vi "Unregister-user-events.vi"(8 "error in (no error)":errorcluster, 10 "Event registration":refnum<event-registration>, 11 "Object ref in":T1) -> (0 "error out":errorcluster, 3 "Object ref out":T1)   [LabVIEW 2013, in "MaterialCharacterization.lvlib" / "MC-Main.lvclass"]
uses:
  MC-Main.lvclass
  Object-reference.ctl
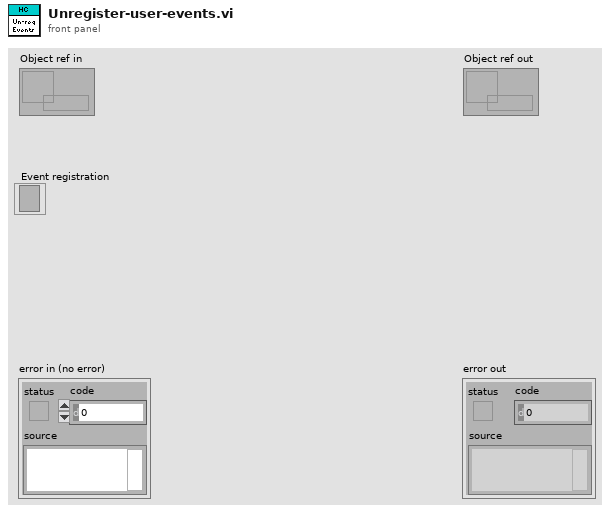
[diagram p1: front panel]
types:
  T1 = typedef "MaterialCharacterization.lvlib/MC-Main.lvclass/Object-reference.ctl" = refnum<data-value>
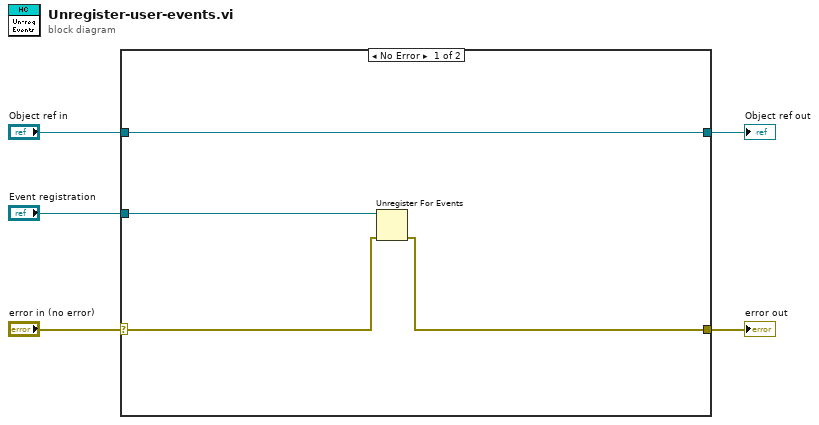
[diagram p0: block diagram]
diagram:
  n1 = case shown="No Error" "error in (no error)" {
    selector: "error in (no error)" -> [w8 w11]
    tunnel: [w7 w11] -> w4
    tunnel: [w9 w10] -> w2
    tunnel: "Object ref in" -> [w9 w10]
    tunnel: "Event registration" -> [w6 _]
    frame No Error {
      n2 = Unregister For Events(event registration refnum=w6, error in=w8) -> (error out=w7:errorcluster)
    }
    frame Error {
    }
  }
  "error out" <- w4
  "Object ref out" <- w2
